vi "initialize needle.vi"(1 "Switch to (A/B)":enum16{"A", "B"}(ring)) -> ()   [LabVIEW 2023]
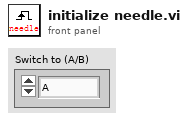
[diagram p1: front panel]
types:
  T1 = enum16{"plate1", "plate2", "plate3", "rinse", "seat"}
  T2 = enum16{"Initialize", "Absolute Position", "Relative Pickup", "Relative Dispense", "Swich valve", "Bypass"}
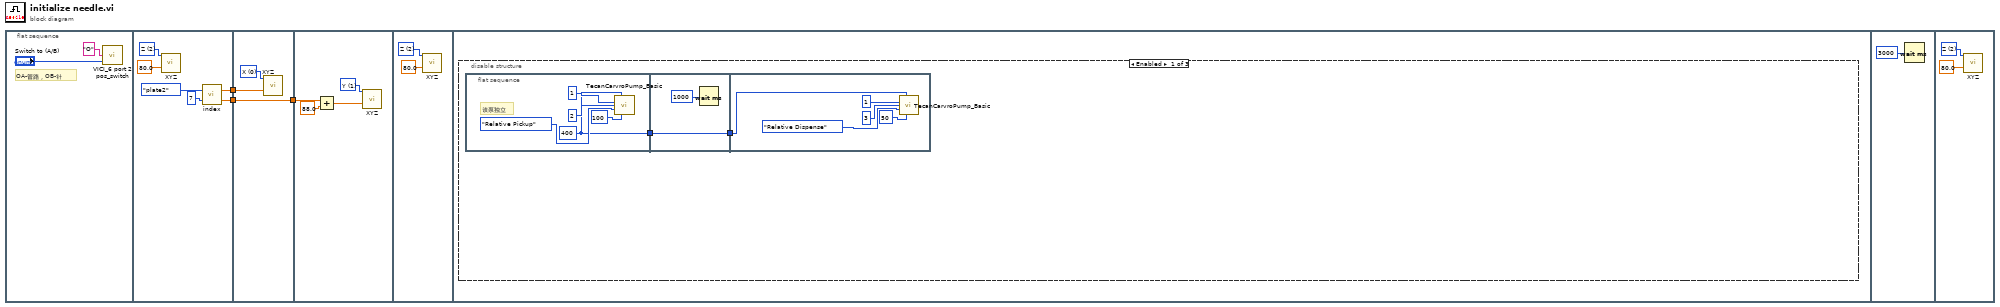
[diagram p0: block diagram]
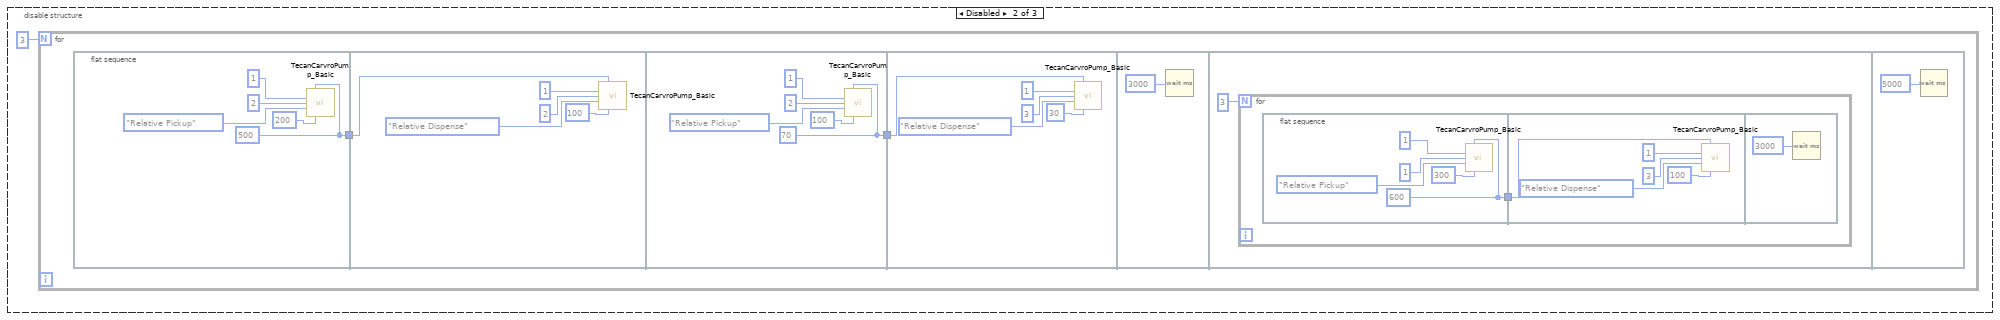
[diagram p2: hidden frame]
diagram:
  n1 = flat-sequence {
    tunnel: [w7] -> w3
    tunnel: [w6] -> w1
    tunnel: w3 -> [w13]
    tunnel: [w12] -> w2
    tunnel: w1 -> [w12]
    tunnel: w2 -> [w17]
    frame #0 {
      # "OA-管路，OB-针"
      n2 = call "VICI_6 port 2 pos_switch.vi"("Switch to position (A/B)"="Switch to (A/B)", "Valve ID"="O") -> ()  [unwired: 2 in, 1 out]
    }
    frame #1 {
      w11 = u16 2 items=["X", "Y", "Z"] ("AXIS")
      n3 = call "XYZ.vi"("AXIS"=w11, "Set location (mm)"=80.0) -> ()  [unwired: 9 in, 5 out]
      n4 = call "index.vi"("index"=i8 7, "where"=T1."plate2") -> ("Y"=w6:dbl, "X"=w7:dbl)
    }
    frame #2 {
      w14 = u16 0 items=["X", "Y", "Z"] ("AXIS")
      n5 = call "XYZ.vi"("AXIS"=w14, "Set location (mm)"=w13) -> ()  [unwired: 9 in, 5 out]
    }
    frame #3 {
      w18 = u16 1 items=["X", "Y", "Z"] ("AXIS")
      n6 = Add(x=w17, y=88.0) -> (x+y=w15:dbl)
      n7 = call "XYZ.vi"("AXIS"=w18, "Set location (mm)"=w15) -> ()  [unwired: 9 in, 5 out]
    }
    frame #4 {
      w20 = u16 2 items=["X", "Y", "Z"] ("AXIS")
      n8 = call "XYZ.vi"("AXIS"=w20, "Set location (mm)"=80.0) -> ()  [unwired: 9 in, 5 out]
    }
    frame #5 {
      n9 = disable-structure shown="Enabled" {
        frame Enabled {
          n10 = flat-sequence {
            tunnel: [w23] -> w22
            tunnel: w22 -> [w29]
            tunnel: [w29] -> w21
            tunnel: w21 -> [w30]
            frame #0 {
              w23 = u16 400 ("Volume (μL)")
              # "该泵独立"
              n11 = call "TecanCarvroPump_Basic.vi"("Volume (μL)"=w23, "TecanPump address"=u8 1, "Valve"=u8 2, "Mode"=T2."Relative Pickup", "Speed (μL/s)"=u16 100) -> ()  [unwired: 10 in, 1 out]
            }
            frame #1 {
              n12 = Wait (ms)(milliseconds to wait=u32 1000) -> ()  [unwired: 1 out]
            }
            frame #2 {
              n13 = call "TecanCarvroPump_Basic.vi"("Volume (μL)"=w30, "TecanPump address"=u8 1, "Valve"=u8 3, "Mode"=T2."Relative Dispense", "Speed (μL/s)"=u16 50) -> ()  [unwired: 10 in, 1 out]
            }
          }
        }
        frame Disabled {
          n14 = for {
            N: 3 -> [_]
            n15 = flat-sequence {
              tunnel: [w38] -> w37
              tunnel: w37 -> [w43]
              tunnel: [w48] -> w36
              tunnel: w36 -> [w53]
              frame #0 {
                w38 = u16 500 ("Volume (μL)")
                n16 = call "TecanCarvroPump_Basic.vi"("Volume (μL)"=w38, "TecanPump address"=u8 1, "Valve"=u8 2, "Mode"=T2."Relative Pickup", "Speed (μL/s)"=u16 200) -> ()  [unwired: 10 in, 1 out]
              }
              frame #1 {
                n17 = call "TecanCarvroPump_Basic.vi"("Volume (μL)"=w43, "TecanPump address"=u8 1, "Valve"=u8 2, "Mode"=T2."Relative Dispense", "Speed (μL/s)"=u16 100) -> ()  [unwired: 10 in, 1 out]
              }
              frame #2 {
                w48 = u16 70 ("Volume (μL)")
                n18 = call "TecanCarvroPump_Basic.vi"("Volume (μL)"=w48, "TecanPump address"=u8 1, "Valve"=u8 2, "Mode"=T2."Relative Pickup", "Speed (μL/s)"=u16 100) -> ()  [unwired: 10 in, 1 out]
              }
              frame #3 {
                n19 = call "TecanCarvroPump_Basic.vi"("Volume (μL)"=w53, "TecanPump address"=u8 1, "Valve"=u8 3, "Mode"=T2."Relative Dispense", "Speed (μL/s)"=u16 30) -> ()  [unwired: 10 in, 1 out]
              }
              frame #4 {
                n20 = Wait (ms)(milliseconds to wait=u32 3000) -> ()  [unwired: 1 out]
              }
              frame #5 {
                n21 = for {
                  N: 3 -> [_]
                  n22 = flat-sequence {
                    tunnel: [w61] -> w60
                    tunnel: w60 -> [w66]
                    frame #0 {
                      w61 = u16 600 ("Volume (μL)")
                      n23 = call "TecanCarvroPump_Basic.vi"("Volume (μL)"=w61, "TecanPump address"=u8 1, "Valve"=u8 1, "Mode"=T2."Relative Pickup", "Speed (μL/s)"=u16 300) -> ()  [unwired: 10 in, 1 out]
                    }
                    frame #1 {
                      n24 = call "TecanCarvroPump_Basic.vi"("Volume (μL)"=w66, "TecanPump address"=u8 1, "Valve"=u8 3, "Mode"=T2."Relative Dispense", "Speed (μL/s)"=u16 100) -> ()  [unwired: 10 in, 1 out]
                    }
                    frame #2 {
                      n25 = Wait (ms)(milliseconds to wait=u32 3000) -> ()  [unwired: 1 out]
                    }
                  }
                }
              }
              frame #6 {
                n26 = Wait (ms)(milliseconds to wait=u32 5000) -> ()  [unwired: 1 out]
              }
            }
          }
        }
        frame Disabled {
        }
      }
    }
    frame #6 {
      n27 = Wait (ms)(milliseconds to wait=u32 3000) -> ()  [unwired: 1 out]
    }
    frame #7 {
      w75 = u16 2 items=["X", "Y", "Z"] ("AXIS")
      n28 = call "XYZ.vi"("AXIS"=w75, "Set location (mm)"=80.0) -> ()  [unwired: 9 in, 5 out]
    }
  }
